vi "Debugging mode dialogue.vi"(7 "Section":string, 9 "Loaded value for \"DevPC - No hardware\"":bool, 11 "Setup.ini ref":T1) -> (3 "Setup.ini ref":T1)   [LabVIEW 2017]
uses:
  <vilib>/Utility/config.llb/Config Data RefNum.ctl
  Global Variables/General Globals.vi
  <vilib>/Utility/config.llb/Write Key (Boolean).vi
  <vilib>/Utility/config.llb/NI_LVConfig.lvlib
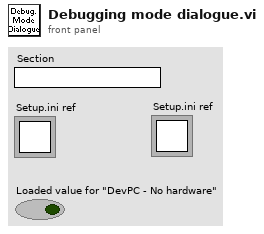
[diagram p1: front panel]
types:
  T1 = typedef "NI_LVConfig.lvlib/Config Data RefNum.ctl" = refnum<k1>
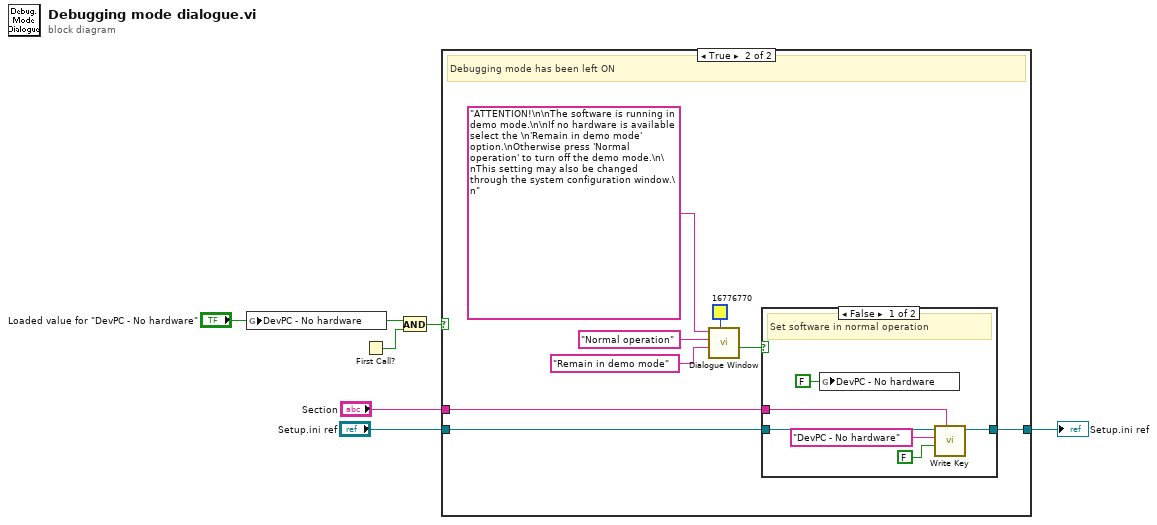
[diagram p0: block diagram]
diagram:
  n1 = global write "General Globals.vi" "DevPC - No hardware"("Loaded value for \"DevPC - No hardware\"") -> ()
  n2 = First Call?() -> (First Call?: T/F=w5:bool)
  n3 = And(x="Loaded value for \"DevPC - No hardware\"", y=w5) -> (x .and. y?=w4:bool)
  n4 = case shown="True" w4 {
    tunnel: [w7 w10] -> w3
    tunnel: "Setup.ini ref" -> [w7 w9]
    tunnel: "Section" -> [_ w8]
    frame False {
      # "Not in demo mode"
    }
    frame True {
      # "Debugging mode has been left ON"
      n5 = call "Dialogue Window.vi"("Colour"=u32 16776770, "Caption-Left button (Cancel)"="Remain in demo mode", "Caption-Right button (OK)"="Normal operation", "Message string"="ATTENTION!\n\nThe software is running in demo mode.\n\nIf no hardware is available select the \n'Remain in demo mode' option.\nOtherwise press 'Normal operation' to turn off the demo mode.\n\nThis setting may also be changed through the system configuration window.\n") -> ("Cancelled (Left button pressed)"=w11:bool)  [unwired: 5 in, 2 out]
      n6 = case shown="False" w11 {
        tunnel: [w19 w22] -> w10
        tunnel: w9 -> [w20 w22]
        tunnel: w8 -> [w17 _]
        frame False {
          # "Set software in normal operation"
          n7 = global write "General Globals.vi" "DevPC - No hardware"(FALSE ("DevPC - No hardware")) -> ()
          n8 = call-poly <vilib>:"Write Key.vi"("section"=w17, "value"=FALSE ("DevPC - No hardware"), "key"="DevPC - No hardware", "refnum"=w20) -> ("refnum out"=w19:T1)  [unwired: 5 in, 2 out]
        }
        frame True {
          # "Keep debugging mode ON"
        }
      }
    }
  }
  "Setup.ini ref" <- w3
